vi "Channel comments.vi"() -> (0 "Comments on channels":string)   [LabVIEW 2013]
uses:
  Lock-in Globals Multiple Inputs and Outputs.vi
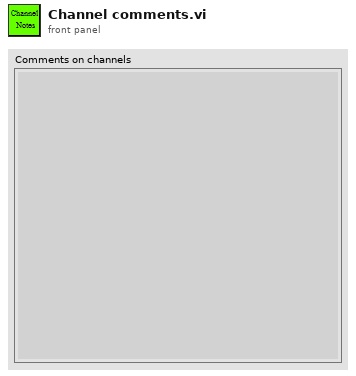
[diagram p1: front panel]
types:
  T1 = cluster{"Signal Type":enum16{"Sine Wave", "Triangle Wave", "Square Wave", "Sawtooth Wave"}, "DC":dbl, "Amplitude":dbl, "frequency":dbl, "Phase":dbl}[]
  T2 = cluster{"Signal Type":enum16{"Sine Wave", "Triangle Wave", "Square Wave", "Sawtooth Wave"}, "DC":dbl, "Amplitude":dbl, "frequency":dbl, "Phase":dbl}
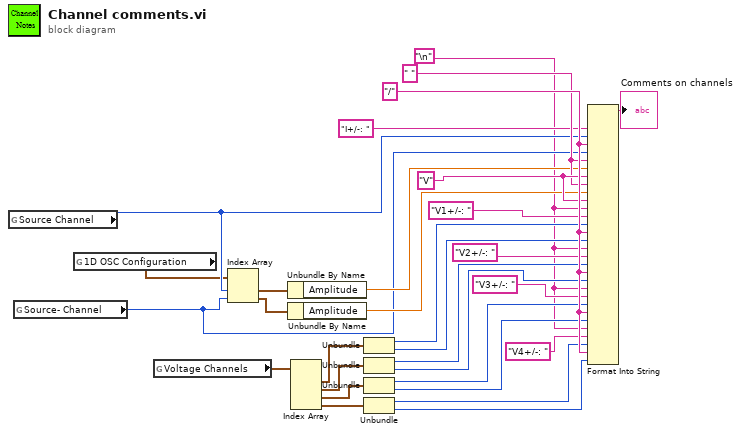
[diagram p0: block diagram]
diagram:
  w1 = "\n"
  w17 = "V"
  w15 = " "
  w29 = "/"
  n1 = global read "Lock-in Globals Multiple Inputs and Outputs.vi" "Source Channel"() -> (w12:i32)
  n2 = global read "Lock-in Globals Multiple Inputs and Outputs.vi" "Source- Channel"() -> (w13:i32)
  n3 = global read "Lock-in Globals Multiple Inputs and Outputs.vi" "1D OSC Configuration"() -> (w10:T1)
  n4 = global read "Lock-in Globals Multiple Inputs and Outputs.vi" "Voltage Channels"() -> (w3:cluster{"V+ Channel":i32, "V- Channel":i32}[])
  n5 = Index Array(array=w10, index #1=w12, index #2=w13) -> (element #1=w9:T2, element #2=w11:T2)
  n6 = Unbundle By Name(w9) -> ("Amplitude"=w14:dbl)
  n7 = Unbundle By Name(w11) -> ("Amplitude"=w16:dbl)
  n8 = Index Array(array=w3) -> (element #1=w4:cluster{"V+ Channel":i32, "V- Channel":i32}, element #2=w5:cluster{"V+ Channel":i32, "V- Channel":i32}, element #3=w6:cluster{"V+ Channel":i32, "V- Channel":i32}, element #4=w7:cluster{"V+ Channel":i32, "V- Channel":i32})  [unwired: 4 in]
  n9 = Unbundle(w4) -> ("V+ Channel"=w19:i32, "V- Channel"=w22:i32)
  n10 = Unbundle(w5) -> ("V+ Channel"=w20:i32, "V- Channel"=w25:i32)
  n11 = Unbundle(w6) -> ("V+ Channel"=w24:i32, "V- Channel"=w26:i32)
  n12 = Unbundle(w7) -> ("V+ Channel"=w28:i32, "V- Channel"=w30:i32)
  n13 = Format Into String("I+/-: ", w12, w29, w13, w15, w14, w17, w15, w16, w17, w1, "V1+/-: ", w19, w29, w22, w1, "V2+/-: ", w20, w29, w25, w1, "V3+/-: ", w24, w29, w26, w1, "V4+/-: ", w28, w29, w30) -> (resulting string=→"Comments on channels":string)  [unwired: 3 in, 1 out]
